vi "Read Status.vi"(8 "Error In":errorcluster, 11 "KIT-QVA in":refnum<class "KIT-QVA.lvclass">) -> (0 "Error Out":errorcluster, 3 "KIT-QVA out":refnum<class "KIT-QVA.lvclass">)   [LabVIEW 2014, in "KIT-QVA.lvlib" / "KIT-QVA.lvclass"]
doc: "Periodically read status of rack, detectors and hardware and publish."
uses:
  KIT-QVA.lvclass
  <vilib>/ActorFramework/Actor/Actor.lvclass/Actor.ctl
  <vilib>/ActorFramework/Message Enqueuer/Message Enqueuer.lvclass/Message Enqueuer.ctl
  <vilib>/ActorFramework/Message Enqueuer/Init from Existing Queue.vi
  <vilib>/ActorFramework/Message Enqueuer/Enqueue.vi
  <vilib>/ActorFramework/Message Priority Queue/Priority Enqueue.vi
  <vilib>/ActorFramework/Message Enqueuer/Message Enqueuer.lvclass
  KIT-QVA Messages/Read Status Msg/Read Status Msg.lvclass
  <vilib>/ActorFramework/Actor/Actor.lvclass
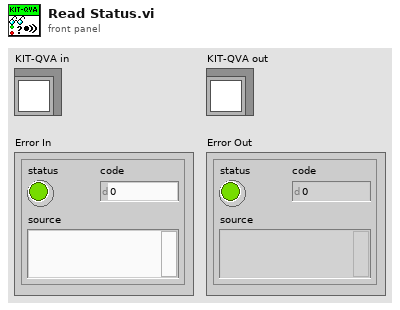
[diagram p1: front panel]
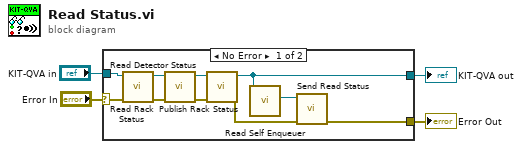
[diagram p0: block diagram]
diagram:
  n1 = case shown="No Error" "Error In" {
    selector: "Error In" -> [w10 w16]
    tunnel: [w6 w16] -> w3
    tunnel: [w8 w15] -> w1
    tunnel: "KIT-QVA in" -> [w9 w15]
    frame No Error {
      n2 = call "Read Rack Status.vi"("Error In"=w10, "KIT-QVA in"=w9) -> ("Error Out"=w11:errorcluster, "KIT-QVA out"=w14:refnum<class "KIT-QVA.lvclass">)  [unwired: 8 in]
      n3 = call "Read Detector Status.vi"("Error In"=w11, "KIT-QVA in"=w14) -> ("Error Out"=w12:errorcluster, "KIT-QVA out"=w13:refnum<class "KIT-QVA.lvclass">)  [unwired: 8 in]
      n4 = call "Publish Rack Status.vi"("Error In"=w12, "KIT-QVA in"=w13) -> ("Error Out"=w7:errorcluster, "KIT-QVA out"=w8:refnum<class "KIT-QVA.lvclass">)  [unwired: 8 in]
      n5 = call <vilib>:"Read Self Enqueuer.vi"("Actor"=w8) -> ("Self Enqueuer"=w5:refnum<class "Message Enqueuer.lvclass">)  [unwired: 10 in]
      n6 = call "Send Read Status.vi"("error in (no error)"=w7, "Message Enqueuer"=w5) -> ("error out"=w6:errorcluster)  [unwired: 8 in, 1 out]
    }
    frame Error {
    }
  }
  "Error Out" <- w3
  "KIT-QVA out" <- w1
